vi "TIFF Check Tile.vi"(6 "para4":cluster{}, 7 "para3":cluster{}, 8 "error in (no error)":errorcluster, 9 "para2":cluster{}, 10 "para1":cluster{}, 11 "para0":cluster{}) -> (0 "error out":errorcluster, 2 "function return":i32, 3 "para0 out":cluster{})   [LabVIEW 2018]
doc: "LIBTIFF_DLL_IMPEXP int TIFFCheckTile(TIFF*, uint32, uint32, uint32, tsample_t);\nextern int TIFFCheckTile(TIFF*, uint32, uint32, uint32, tsample_t);"
uses:
  libtiff3.dll
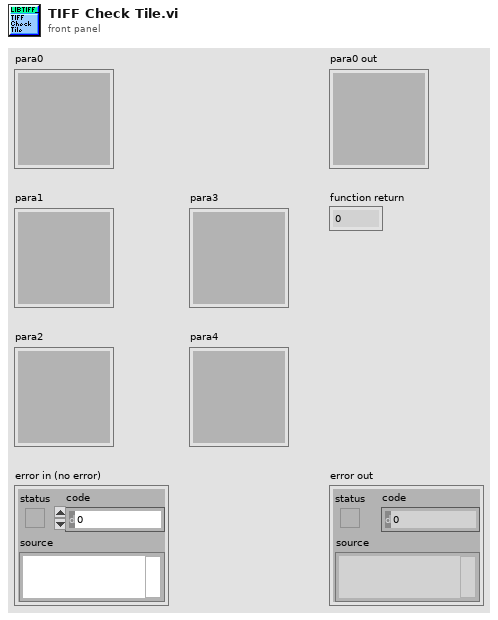
[diagram p1: front panel]
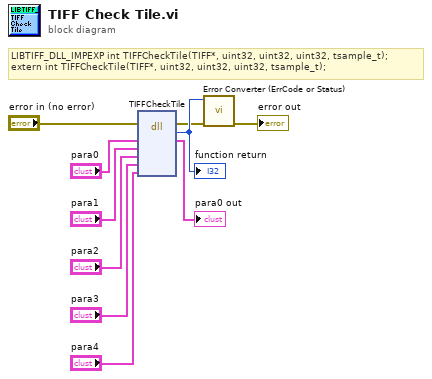
[diagram p0: block diagram]
diagram:
  # "LIBTIFF_DLL_IMPEXP\tint TIFFCheckTile(TIFF*, uint32, uint32, uint32, tsample_t);\nextern\tint TIFFCheckTile(TIFF*, uint32, uint32, uint32, tsample_t);"
  n1 = dll-call lib="C:/Users/johan/Downloads/LabVIEW software/LabVIEW software/IX-81 Software/lib/tiff/LibTiffLabview/libtiff3.*" fn="TIFFCheckTile"(error in="error in (no error)", "para0"="para0", "para1"="para1", "para2"="para2", "para3"="para3", "para4"="para4") -> (error out=w2:errorcluster, w10:i32, "para0"=→"para0 out":cluster{})  [unwired: 6 in, 1 out]
  "function return" <- w10
  n2 = call "Error Converter (ErrCode or Status).vi"("error in (no error)"=w2, "error code"=w10) -> ("error out"=→"error out":errorcluster)  [unwired: 9 in]
